vi "FG-Open-config.vi"(8 "error in":errorcluster, 10 "Storage params":refnum<data-value>, 11 "Config. params. ref. in":refnum<data-value>) -> (0 "error IO":errorcluster, 3 "Config. params. ref.":refnum<data-value>)   [LabVIEW 2013, in "CameraVision.lvlib" / "CV-Configuration.lvclass"]
uses:
  CV-Configuration.lvclass
  Storage/CV-Storage.lvclass
  Storage/CV-Storage.lvclass/CV-Storage.ctl
  CV-Configuration.lvclass/CV-Configuration.ctl
  Storage/Read Base path.vi
  Read Framegrabber DLL file.vi
  Read Framegrabber board.vi
  Write BoardHandle.vi
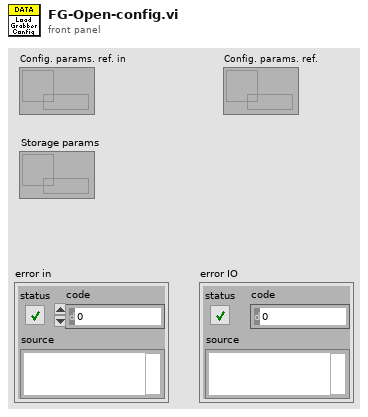
[diagram p1: front panel]
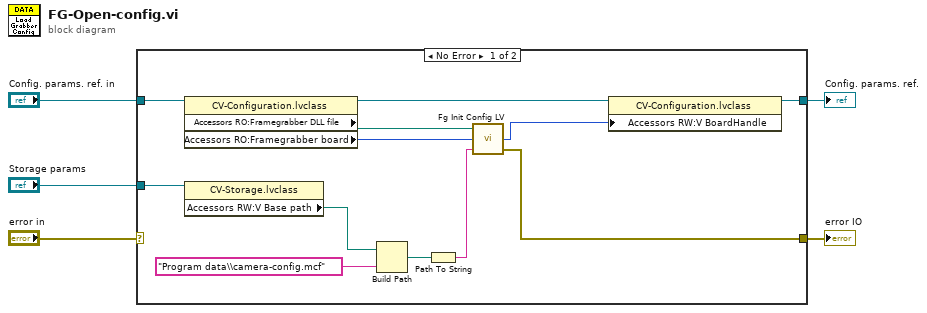
[diagram p0: block diagram]
diagram:
  n1 = case shown="No Error" "error in" {
    selector: "error in" -> [_ w19]
    tunnel: [w8 w19] -> w5
    tunnel: "Config. params. ref. in" -> [w17 w18]
    tunnel: [w15 w18] -> w2
    tunnel: "Storage params" -> [w7 _]
    frame No Error {
      n2 = property class="CV-Configuration.lvclass"(reference=w17) -> (reference out=w16:refnum<data-value>, "Accessors RO:Framegrabber DLL file"=w12:path, "Accessors RO:Framegrabber board"=w13:i32)  [unwired: 1 in, 1 out]
      n3 = property class="CV-Storage.lvclass"(reference=w7) -> ("Accessors RW:V Base path"=w6:path)  [unwired: 1 in, 2 out]
      n4 = Build Path(base path=w6, name or relative path="Program data\\camera-config.mcf") -> (appended path=w10:path)
      n5 = Path To String(path=w10) -> (string=w14:string)
      n6 = call <userlib>:"Fg Init Config LV.vi"("Config_Name"=w14, "NumberOfmEnable"=w13, "dll path in"=w12) -> ("error out"=w8:errorcluster, "function return"=w11:u64)  [unwired: 1 out]
      n7 = property class="CV-Configuration.lvclass"(reference=w16, "Accessors RW:V BoardHandle"=w11) -> (reference out=w15:refnum<data-value>)  [unwired: 1 in, 1 out]
    }
    frame Error {
    }
  }
  "error IO" <- w5
  "Config. params. ref." <- w2
